vi "Pos_or_Neg.vi"() -> ()   [LabVIEW 2025]
panel:
  out "Result":string
  in  "X":dbl
  # "Result = x/2 - 10"
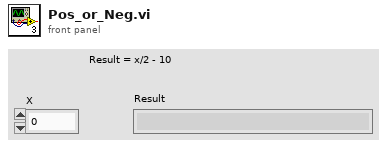
[diagram p1: front panel]
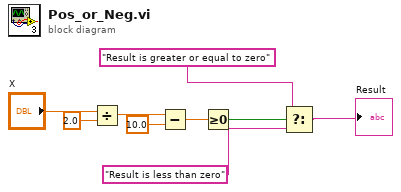
[diagram p0: block diagram]
diagram:
  n1 = Divide(x="X", y=2.0) -> (x/y=w7:dbl)
  n2 = Subtract(x=w7, y=10.0) -> (x-y=w4:dbl)
  n3 = Greater Or Equal To 0?(x=w4) -> (x >= 0?=w5:bool)
  n4 = Select(t="Result is greater or equal to zero", s=w5, f="Result is less than zero") -> (s? t:f=→"Result":string)
